vi "Climb Status.vi"(11 "Climb Status Cluster":T1) -> (1 "Color Box":u32, 2 "Blink":bool, 3 "Value":string)   [LabVIEW 2017]
uses:
  Common Code/Climb Status Cluster.ctl
panel:
  in  "Iterations":dbl
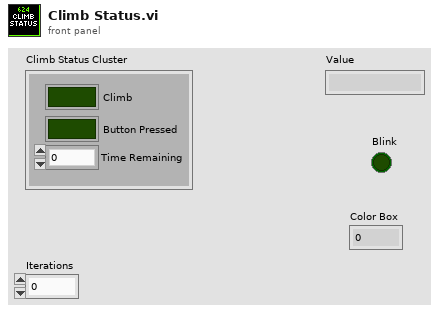
[diagram p1: front panel]
types:
  T1 = typedef "Climb Status Cluster.ctl" = cluster{"Climb":bool, "Button Pressed":bool, "Time Remaining":dbl}
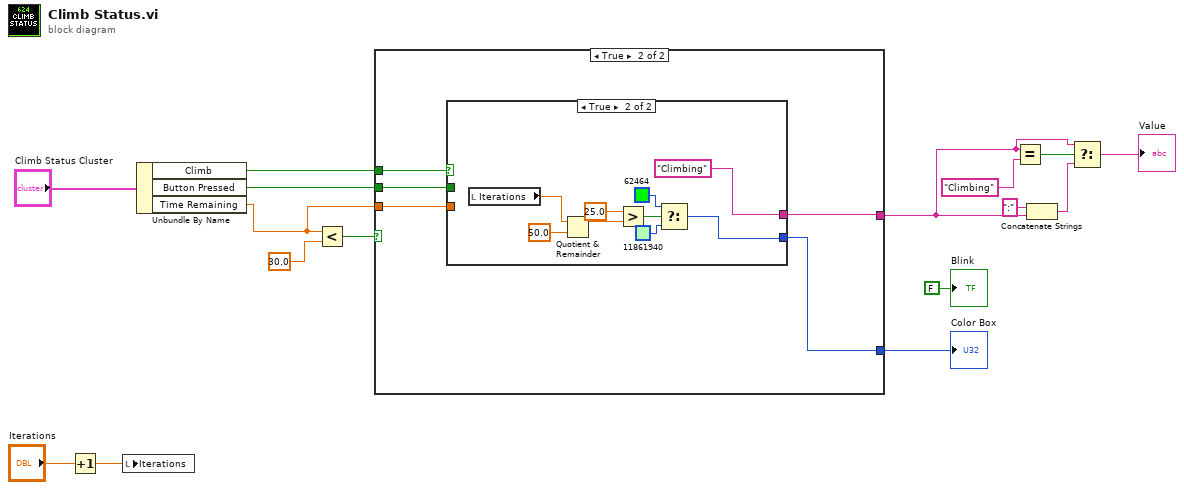
[diagram p0: block diagram]
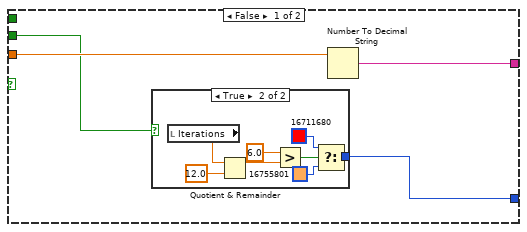
[diagram p2: hidden frame]
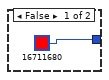
[diagram p3: hidden frame]
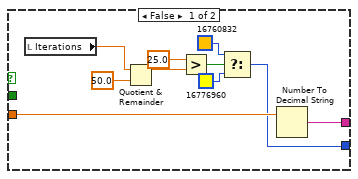
[diagram p4: hidden frame]
diagram:
  n1 = Increment(x="Iterations") -> (x+1=w9:dbl)
  n2 = local write "Iterations"(w9) -> ()
  n3 = Unbundle By Name("Climb Status Cluster") -> ("Climb"=w10:bool, "Button Pressed"=w12:bool, "Time Remaining"=w13:dbl)
  n4 = Less?(x=w13, y=30.0) -> (x < y?=w15:bool)
  n5 = case shown="True" w15 {
    tunnel: w13 -> [w20 w33]
    tunnel: w12 -> [w17 w30]
    tunnel: w10 -> [_ w34]
    tunnel: [w19 w32] -> w3
    tunnel: [w18 w31] -> w11
    frame False {
      n6 = case shown="True" w17 {
        tunnel: [u32 16711680 ("Color Box") w24] -> w18
        frame False {
        }
        frame True {
          n7 = local read "Iterations"() -> (w22:dbl)
          n8 = Quotient & Remainder(x=w22, y=12.0) -> (x-y*floor(x/y)=w29:dbl)  [unwired: 1 out]
          n9 = Greater?(x=6.0, y=w29) -> (0:w26:bool)
          n10 = Select(t=u32 16711680 ("Color Box"), s=w26, f=u32 16755801 ("Color Box")) -> (s? t:f=w24:u32)
        }
      }
      n11 = Number To Decimal String(number=w20) -> (decimal integer string=w19:string)  [unwired: 1 in]
    }
    frame True {
      n12 = case shown="True" w34 {
        tunnel: w33 -> [w44 _]
        tunnel: [w43 "Climbing"] -> w32
        tunnel: [w35 w46] -> w31
        tunnel: w30 -> [_ _]
        frame False {
          n13 = local read "Iterations"() -> (w40:dbl)
          n14 = Quotient & Remainder(x=w40, y=50.0) -> (x-y*floor(x/y)=w42:dbl)  [unwired: 1 out]
          n15 = Greater?(x=25.0, y=w42) -> (0:w38:bool)
          n16 = Select(t=u32 16760832 ("Color Box"), s=w38, f=u32 16776960 ("Color Box")) -> (s? t:f=w35:u32)
          n17 = Number To Decimal String(number=w44) -> (decimal integer string=w43:string)  [unwired: 1 in]
        }
        frame True {
          n18 = local read "Iterations"() -> (w45:dbl)
          n19 = Quotient & Remainder(x=w45, y=50.0) -> (x-y*floor(x/y)=w52:dbl)  [unwired: 1 out]
          n20 = Greater?(x=25.0, y=w52) -> (0:w49:bool)
          n21 = Select(t=u32 62464 ("Color Box"), s=w49, f=u32 11861940 ("Color Box")) -> (s? t:f=w46:u32)
        }
      }
    }
  }
  "Color Box" <- w11
  n22 = Equal?(x=w3, y="Climbing") -> (x = y?=w5:bool)
  n23 = Concatenate Strings(":" ("string"), w3) -> (w4:string)
  n24 = Select(t=w3, s=w5, f=w4) -> (s? t:f=→"Value":string)
  "Blink" <- FALSE
